vi "Do.vi"(8 "error in (no error)":errorcluster, 10 "Actor in":refnum<class "Actor.lvclass">, 11 "Sample Actor Data Msg":refnum<class "Sample Actor Data Msg.lvclass">) -> (0 "error out":errorcluster, 2 "Actor out":refnum<class "Actor.lvclass">)   [LabVIEW 2016, in "Sample Actor Data Msg.lvclass"]
doc: "(<B>Filename</B>: Actor Framework.lvlib:Message.lvclass:Do.vi)\n\nDefines what a message does when it is received by an actor. Generally, a message instructs an actor to invoke one of its methods. By default, this method does nothing. A child class must override it to define behavior. Create a child class by using the Actor Framework Message Maker dialog box.\n\n--\nCopyright © 2017 Composed SystemsI All rights reserved.\n\nAuthor: Jon McBee <jon.mcbee@composed.io>\n\nThis library is provided \"AS IS\" ,WITHOUT WARRANTIES OR\nCONDITIONS OF ANY KIND, either express or implied.\n\nComposed Systems -- composed.io\n\nStream 0.0.1.1\nJon McBee - Composed Systems\nCopyright (c) 2017, Composed Systems"
uses:
  <userlib>/Composed Systems/Stream/Mediator/Example/Example Actor Messages/Sample Actor Data Msg/Sample Actor Data Msg.lvclass
  C:/Program Files (x86)/National Instruments/LabVIEW 2016/user.lib/Composed Systems/Stream/Mediator/Classes/Message AF Mediator/Message AF Mediator.lvclass
  <vilib>/ActorFramework/Actor/Actor.lvclass
  <userlib>/Composed Systems/Stream/Mediator/Example/Example Actor/Example Actor.lvclass
  C:/Program Files (x86)/National Instruments/LabVIEW 2016/vi.lib/ActorFramework/Actor/Actor.lvclass
  <userlib>/Composed Systems/Stream/Mediator/Classes/Message Double/Message Double.lvclass
  <userlib>/Composed Systems/Stream/Mediator/Classes/Message AF Mediator/Message AF Mediator.lvclass
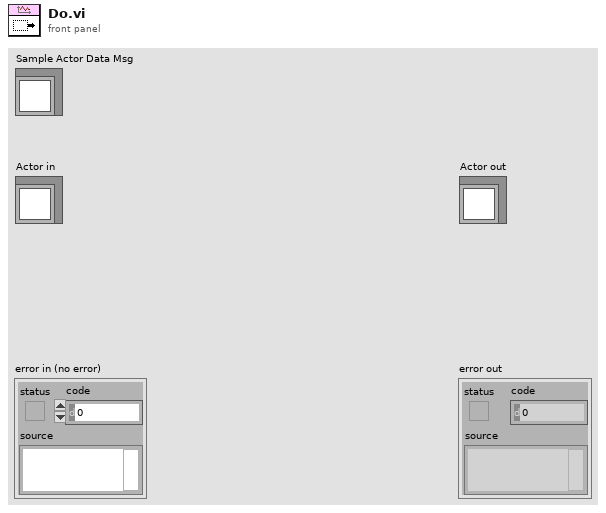
[diagram p1: front panel]
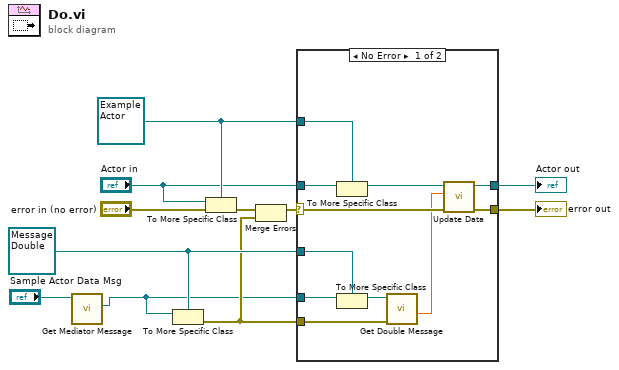
[diagram p0: block diagram]
diagram:
  w4 = refnum<class "Message Double.lvclass"> refnum ("Message Double.lvclass")
  w10 = refnum<class "Example Actor.lvclass"> refnum ("Example Actor.lvclass")
  n1 = call <userlib>:"Get Mediator Message.vi"("Message AF Mediator in"="Sample Actor Data Msg") -> ("Mediator Message"=w1:refnum<class "Message Interface.lvclass">)  [unwired: 8 in, 2 out]
  n2 = To More Specific Class(target class=w4, reference=w1) -> (error out=w3:errorcluster)  [unwired: 1 in, 1 out]
  n3 = To More Specific Class(target class=w10, reference="Actor in", error in="error in (no error)") -> (error out=w11:errorcluster)  [unwired: 1 out]
  n4 = Merge Errors(w11, w3) -> (w5:errorcluster)
  n5 = case shown="No Error" w5 {
    selector: w5 -> [w19 w23]
    tunnel: w10 -> [w20 _]
    tunnel: "Actor in" -> [w22 w24]
    tunnel: [w18 w24] -> w8
    tunnel: [w17 w23] -> w7
    tunnel: w1 -> [w16 _]
    tunnel: w4 -> [w15 _]
    tunnel: w3 -> [w13 _]
    frame No Error {
      n6 = To More Specific Class(target class=w20, reference=w22) -> (specific class reference=w21:refnum<class "Example Actor.lvclass">)  [unwired: 1 in, 1 out]
      n7 = To More Specific Class(target class=w15, reference=w16) -> (specific class reference=w14:refnum<class "Message Double.lvclass">)  [unwired: 1 in, 1 out]
      n8 = call <userlib>:"Get Double Message.vi"("error in (no error)"=w13, "Message Double in"=w14) -> ("Value"=w12:dbl)  [unwired: 6 in, 3 out]
      n9 = call <userlib>:"Update Data.vi"("error in (no error)"=w19, "Data"=w12, "Example Actor in"=w21) -> ("error out"=w17:errorcluster, "Example Actor out"=w18:refnum<class "Example Actor.lvclass">)  [unwired: 7 in]
    }
    frame Error {
    }
  }
  "error out" <- w7
  "Actor out" <- w8
